vi "1B_AnalyzeAmplitudeRamp_LimitsGraph.vi"(0 "Target P1":dbl[](array[numeric])=[0.0022, 0.003293999862670899, 0.004371999931335449, 0.0054809996604919435, 0.006590999794006348, 0.0077, 0.00990300006866455], 1 "Target P2":dbl[](array[numeric])=[0.0017600000000000003, 0.002635199890136719, 0.0034975999450683596, 0.004384799728393555, 0.005272799835205079, 0.0061600000000000005, 0.00792240005493164], 2 "Target P3":dbl[](array[numeric])=[0.0011, 0.0016469999313354494, 0.0021859999656677247, 0.0027404998302459718, 0.003295499897003174, 0.00385, 0.004951500034332275], 3 "Target P4":dbl[](array[numeric])=[0.00044000000000000007, 0.0006587999725341798, 0.0008743999862670899, 0.0010961999320983887, 0.0013181999588012696, 0.0015400000000000001, 0.00198060001373291], 6 "Trimmed Elapsed time from Active Stim ( sec )":dbl[](array[numeric])=[1.8767312026320724, 2.978631206395221, 4.068465751042822, 5.166899951203959, 6.281533743458567, 7.396964385960018, 8.492272259914898, 9.593095214062487, 10.689171075006016] format="%#.1g", 7 "Meas. P 1":dbl[](array[numeric])=[0.0018943920703614388, 0.0030743708276341373, 0.004258429367963039, 0.005437393299148003, 0.006592488458447496, 0.007901789494661983, 0.01005856433850231], 8 "Tol [ A ]":dbl=0.0009 format="%#.3p", 9 "Meas. P 2":dbl[](array[numeric])=[0.0018864095105808184, 0.003085641595243711, 0.003400347021083947, 0.004347957724400547, 0.00526950062579862, 0.006319564654557489, 0.008032593675745206], 11 "Meas. P 3":dbl[](array[numeric])=[0.0015041390106394037, 0.0024611423149691505, 0.002128203324710528, 0.0027220654544606523, 0.0032842044427856365, 0.003946290566028238, 0.005010347737121928], 13 "Meas. P 4":dbl[](array[numeric])=[0.0007465336063221649, 0.0011622407406179668, 0.0008495359928646463, 0.0010947535709027161, 0.0013074604950968907, 0.0015731887719878195, 0.0019857310368747907]) -> (17 "P1 mean error [ A ]":dbl format="%#.0p")   [LabVIEW 2010]
panel:
  out "P4":cluster{dbl[], dbl[]}[](graph)=[{[1.8767312026320724, 2.978631206395221, 4.068465751042822, 5.166899951203959, 6.281533743458567, 7.396964385960018, 8.492272259914898, 9.593095214062487, 10.689171075006016], [0.0022, 0.003293999862670899, 0.004371999931335449, 0.0054809996604919435, 0.006590999794006348, 0.0077, 0.00990300006866455]}, {[1.8767312026320724, 2.978631206395221, 4.068465751042822, 5.166899951203959, 6.281533743458567, 7.396964385960018, 8.492272259914898, 9.593095214062487, 10.689171075006016], [0.0031000000000000003, 0.004193999862670899, 0.005271999931335449, 0.006380999660491943, 0.007490999794006348, 0.0086, 0.01080300006866455]}, {[1.8767312026320724, 2.978631206395221, 4.068465751042822, 5.166899951203959, 6.281533743458567, 7.396964385960018, 8.492272259914898, 9.593095214062487, 10.689171075006016], [0.0013000000000000002, 0.002393999862670899, 0.0034719999313354497, 0.004580999660491944, 0.005690999794006348, 0.0068000000000000005, 0.00900300006866455]}, {[1.8767312026320724, 2.978631206395221, 4.068465751042822, 5.166899951203959, 6.281533743458567, 7.396964385960018, 8.492272259914898, 9.593095214062487, 10.689171075006016], [0.0018943920703614388, 0.0030743708276341373, 0.004258429367963039, 0.005437393299148003, 0.006592488458447496, 0.007901789494661983, 0.01005856433850231]}]
  out "P3":cluster{dbl[], dbl[]}[](graph)=[{[1.8767312026320724, 2.978631206395221, 4.068465751042822, 5.166899951203959, 6.281533743458567, 7.396964385960018, 8.492272259914898, 9.593095214062487, 10.689171075006016], [0.0022, 0.003293999862670899, 0.004371999931335449, 0.0054809996604919435, 0.006590999794006348, 0.0077, 0.00990300006866455]}, {[1.8767312026320724, 2.978631206395221, 4.068465751042822, 5.166899951203959, 6.281533743458567, 7.396964385960018, 8.492272259914898, 9.593095214062487, 10.689171075006016], [0.0031000000000000003, 0.004193999862670899, 0.005271999931335449, 0.006380999660491943, 0.007490999794006348, 0.0086, 0.01080300006866455]}, {[1.8767312026320724, 2.978631206395221, 4.068465751042822, 5.166899951203959, 6.281533743458567, 7.396964385960018, 8.492272259914898, 9.593095214062487, 10.689171075006016], [0.0013000000000000002, 0.002393999862670899, 0.0034719999313354497, 0.004580999660491944, 0.005690999794006348, 0.0068000000000000005, 0.00900300006866455]}, {[1.8767312026320724, 2.978631206395221, 4.068465751042822, 5.166899951203959, 6.281533743458567, 7.396964385960018, 8.492272259914898, 9.593095214062487, 10.689171075006016], [0.0018943920703614388, 0.0030743708276341373, 0.004258429367963039, 0.005437393299148003, 0.006592488458447496, 0.007901789494661983, 0.01005856433850231]}]
  out "P2":cluster{dbl[], dbl[]}[](graph)=[{[1.8767312026320724, 2.978631206395221, 4.068465751042822, 5.166899951203959, 6.281533743458567, 7.396964385960018, 8.492272259914898, 9.593095214062487, 10.689171075006016], [0.0022, 0.003293999862670899, 0.004371999931335449, 0.0054809996604919435, 0.006590999794006348, 0.0077, 0.00990300006866455]}, {[1.8767312026320724, 2.978631206395221, 4.068465751042822, 5.166899951203959, 6.281533743458567, 7.396964385960018, 8.492272259914898, 9.593095214062487, 10.689171075006016], [0.0031000000000000003, 0.004193999862670899, 0.005271999931335449, 0.006380999660491943, 0.007490999794006348, 0.0086, 0.01080300006866455]}, {[1.8767312026320724, 2.978631206395221, 4.068465751042822, 5.166899951203959, 6.281533743458567, 7.396964385960018, 8.492272259914898, 9.593095214062487, 10.689171075006016], [0.0013000000000000002, 0.002393999862670899, 0.0034719999313354497, 0.004580999660491944, 0.005690999794006348, 0.0068000000000000005, 0.00900300006866455]}, {[1.8767312026320724, 2.978631206395221, 4.068465751042822, 5.166899951203959, 6.281533743458567, 7.396964385960018, 8.492272259914898, 9.593095214062487, 10.689171075006016], [0.0018943920703614388, 0.0030743708276341373, 0.004258429367963039, 0.005437393299148003, 0.006592488458447496, 0.007901789494661983, 0.01005856433850231]}]
  out "P1":cluster{dbl[], dbl[]}[](graph)=[{[1.8767312026320724, 2.978631206395221, 4.068465751042822, 5.166899951203959, 6.281533743458567, 7.396964385960018, 8.492272259914898, 9.593095214062487, 10.689171075006016], [0.0022, 0.003293999862670899, 0.004371999931335449, 0.0054809996604919435, 0.006590999794006348, 0.0077, 0.00990300006866455]}, {[1.8767312026320724, 2.978631206395221, 4.068465751042822, 5.166899951203959, 6.281533743458567, 7.396964385960018, 8.492272259914898, 9.593095214062487, 10.689171075006016], [0.0031000000000000003, 0.004193999862670899, 0.005271999931335449, 0.006380999660491943, 0.007490999794006348, 0.0086, 0.01080300006866455]}, {[1.8767312026320724, 2.978631206395221, 4.068465751042822, 5.166899951203959, 6.281533743458567, 7.396964385960018, 8.492272259914898, 9.593095214062487, 10.689171075006016], [0.0013000000000000002, 0.002393999862670899, 0.0034719999313354497, 0.004580999660491944, 0.005690999794006348, 0.0068000000000000005, 0.00900300006866455]}, {[1.8767312026320724, 2.978631206395221, 4.068465751042822, 5.166899951203959, 6.281533743458567, 7.396964385960018, 8.492272259914898, 9.593095214062487, 10.689171075006016], [0.0018943920703614388, 0.0030743708276341373, 0.004258429367963039, 0.005437393299148003, 0.006592488458447496, 0.007901789494661983, 0.01005856433850231]}]
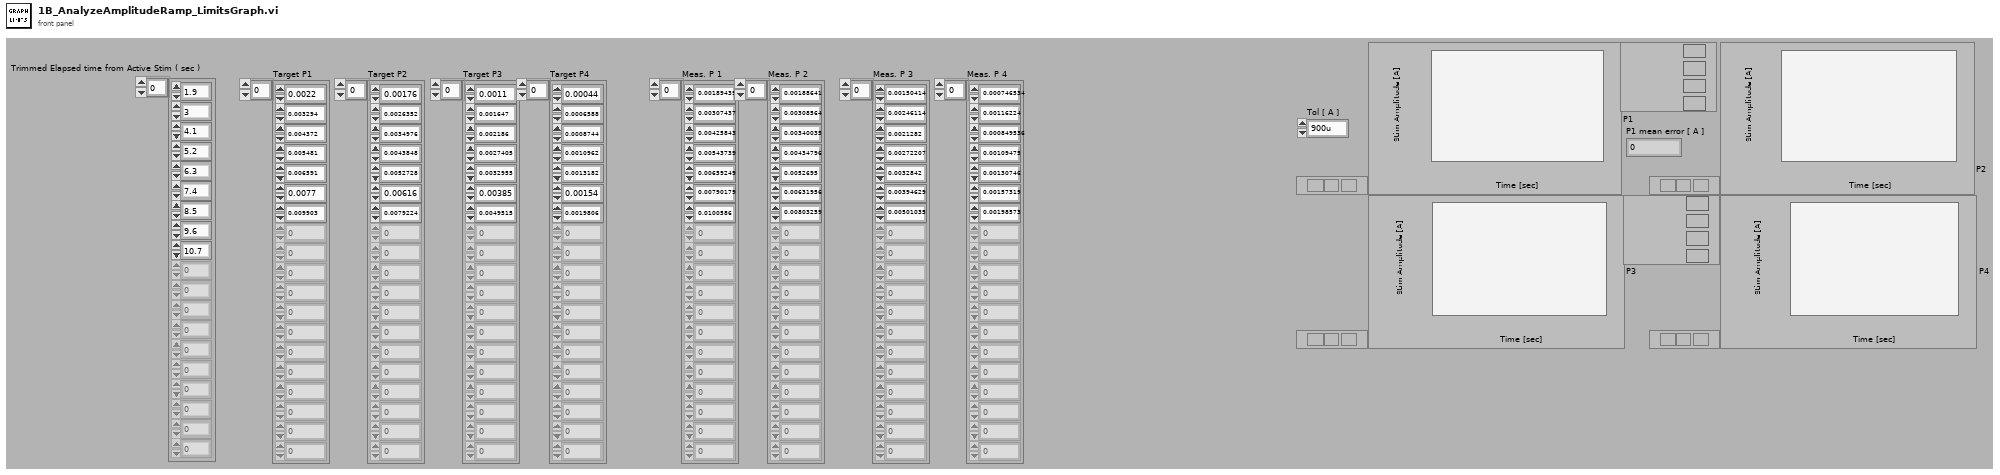
[diagram p1: front panel]
types:
  T1 = cluster{"Trimmed Elapsed time from Active Stim ( sec )":dbl[], "Target P1":dbl[]}[]
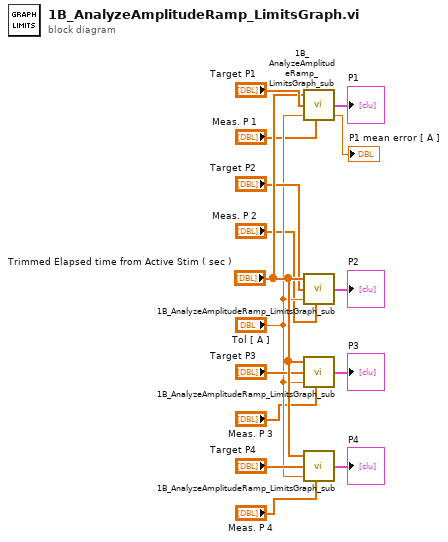
[diagram p0: block diagram]
diagram:
  n1 = call "1B_AnalyzeAmplitudeRamp_LimitsGraph_sub.vi"("Trimmed Elapsed time from Active Stim ( sec )"="Trimmed Elapsed time from Active Stim ( sec )", "Target"="Target P1", "Tol [ A ]"="Tol [ A ]", "Meas."="Meas. P 1") -> ("Array"=→"P1":T1, "mean error"=→"P1 mean error [ A ]":dbl)  [unwired: 4 in]
  n2 = call "1B_AnalyzeAmplitudeRamp_LimitsGraph_sub.vi"("Trimmed Elapsed time from Active Stim ( sec )"="Trimmed Elapsed time from Active Stim ( sec )", "Target"="Target P2", "Tol [ A ]"="Tol [ A ]", "Meas."="Meas. P 2") -> ("Array"=→"P2":T1)  [unwired: 4 in, 1 out]
  n3 = call "1B_AnalyzeAmplitudeRamp_LimitsGraph_sub.vi"("Trimmed Elapsed time from Active Stim ( sec )"="Trimmed Elapsed time from Active Stim ( sec )", "Target"="Target P3", "Tol [ A ]"="Tol [ A ]", "Meas."="Meas. P 3") -> ("Array"=→"P3":T1)  [unwired: 4 in, 1 out]
  n4 = call "1B_AnalyzeAmplitudeRamp_LimitsGraph_sub.vi"("Trimmed Elapsed time from Active Stim ( sec )"="Trimmed Elapsed time from Active Stim ( sec )", "Target"="Target P4", "Tol [ A ]"="Tol [ A ]", "Meas."="Meas. P 4") -> ("Array"=→"P4":T1)  [unwired: 4 in, 1 out]
